vi "DHE_GetMinExpTime.vi"() -> (2 "MinExpTime":sgl)   [LabVIEW 2016]
uses:
  private/vis/DHE_VarAction.ctl
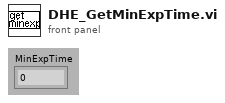
[diagram p1: front panel]
types:
  T1 = typedef "DHE_VarAction.ctl" = enum16{"read", "write"}
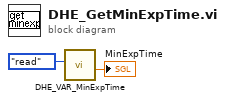
[diagram p0: block diagram]
diagram:
  n1 = call "DHE_VAR_MinExpTime.vi"("action"=DHE_VarAction."read") -> ("MinExpTime"=→"MinExpTime":sgl)  [unwired: 1 in, 9 out]
